vi "7495Test.vi"() -> ()   [LabVIEW 2012]
panel:
  out "Clk1":bool
  out "Clk2":bool
  out "T0 2":bool
  out "T1 2":bool
  out "T2 2":bool
  out "T3 2":bool
  out "T4 2":bool
  out "T5 2":bool
  out "T6 2":bool
  out "T7 2":bool
  out "T7":bool
  out "T6":bool
  out "T5":bool
  out "T4":bool
  out "T3":bool
  out "T2":bool
  out "T1":bool
  out "T0":bool
  out "CT":bool
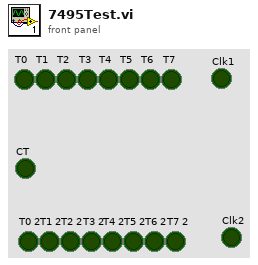
[diagram p1: front panel]
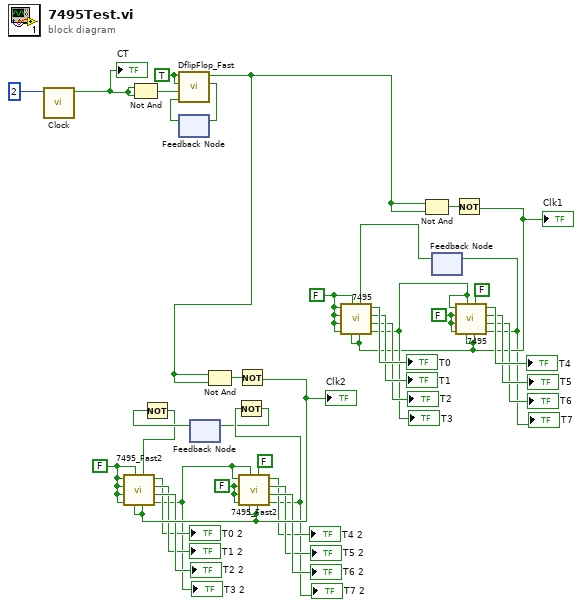
[diagram p0: block diagram]
diagram:
  w9 = FALSE ("B")
  w8 = FALSE ("Mode\nControl")
  w32 = FALSE ("B")
  w33 = FALSE ("Mode\nControl")
  w36 = TRUE ("Set")
  n1 = call "Clock.vi"("Slices"=u32 2) -> ("Clk"=w21:bool)  [unwired: 10 in]
  "CT" <- w21
  n2 = Not And(1:w21, 2:w21) -> (0:w37:bool)
  n3 = feedback #1() -> (w35:bool)  [unwired: 1 in]
  n4 = call "DflipFlop_Fast.vi"("D"=w35, "Clock"=w37, "Reset"=w36, "Set"=w36) -> ("/Q\\"=w30:bool, "Q"=w6:bool)  [unwired: 6 in]
  n5 = feedback-in #1(w30) -> ()
  n6 = feedback #2() -> (w2:bool)  [unwired: 1 in]
  n7 = Not(x=w2) -> (.not. x?=w1:bool)
  n8 = Not And(1:w6, 2:w6) -> (0:w7:bool)
  n9 = Not(x=w7) -> (.not. x?=w17:bool)
  "Clk2" <- w17
  n10 = call "7495_Fast2.vi"("Clk 1\nR-Shift"=w17, "Serial\nInput"=w1, "Clk 2\nL-Shift"=w17, "Mode\nControl"=w8, "D"=w8, "C"=w8, "B"=w8, "A"=w8) -> ("OD"=w5:bool, "OC"=→"T2 2":bool, "OB"=→"T1 2":bool, "OA"=→"T0 2":bool)
  "T3 2" <- w5
  n11 = call "7495_Fast2.vi"("Clk 1\nR-Shift"=w17, "Serial\nInput"=FALSE ("Serial\nInput"), "Clk 2\nL-Shift"=w17, "Mode\nControl"=w5, "D"=w9, "C"=w9, "B"=w9, "A"=w5) -> ("OD"=w4:bool, "OC"=→"T6 2":bool, "OB"=→"T5 2":bool, "OA"=→"T4 2":bool)
  "T7 2" <- w4
  n12 = Not(x=w4) -> (.not. x?=w3:bool)
  n13 = feedback-in #2(w3) -> ()
  n14 = Not And(1:w6, 2:w6) -> (0:w34:bool)
  n15 = feedback #3() -> (w19:bool)  [unwired: 1 in]
  n16 = Not(x=w34) -> (.not. x?=w20:bool)
  "Clk1" <- w20
  n17 = call "7495.vi"("Clk 1\nR-Shift"=w20, "Serial\nInput"=w19, "Clk 2\nL-Shift"=w20, "Mode\nControl"=w33, "D"=w33, "C"=w33, "B"=w33, "A"=w33) -> ("OD"=w25:bool, "OC"=→"T2":bool, "OB"=→"T1":bool, "OA"=→"T0":bool)
  "T3" <- w25
  n18 = call "7495.vi"("Clk 1\nR-Shift"=w20, "Serial\nInput"=FALSE ("Serial\nInput"), "Clk 2\nL-Shift"=w20, "Mode\nControl"=w25, "D"=w32, "C"=w32, "B"=w32, "A"=w25) -> ("OD"=w18:bool, "OC"=→"T6":bool, "OB"=→"T5":bool, "OA"=→"T4":bool)
  "T7" <- w18
  n19 = feedback-in #3(w18) -> ()
